vi "Error Handler.vi"() -> ()   [LabVIEW 2019]
uses:
  <vilib>/Utility/error.llb/Error Cluster From Error Code.vi
  <vilib>/ErrorRing/Error Ring.xnode
panel:
  in  "error in (no error)":errorcluster
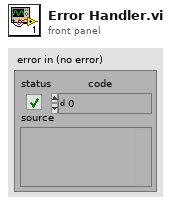
[diagram p1: front panel]
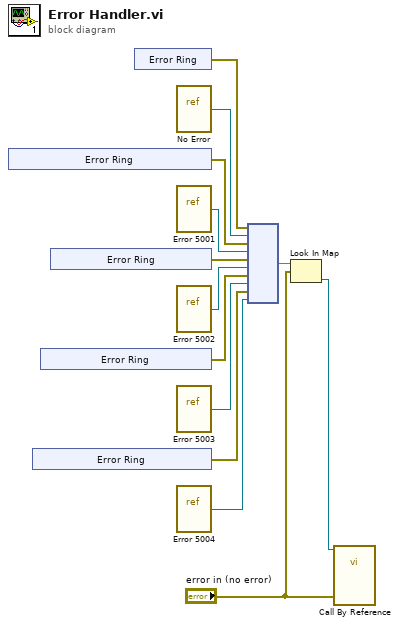
[diagram p0: block diagram]
diagram:
  n1 = xnode "Error Ring"() -> ("error out"=w12:errorcluster)
  n2 = xnode "Error Ring"() -> ("error out"=w6:errorcluster)
  n3 = xnode "Error Ring"() -> ("error out"=w8:errorcluster)
  n4 = xnode "Error Ring"() -> ("error out"=w11:errorcluster)
  n5 = xnode "Error Ring"() -> ("error out"=w13:errorcluster)
  n6 = vi-ref "No Error.vi"() -> (w3:refnum<vi>)
  n7 = vi-ref "Error 5001.vi"() -> (w10:refnum<vi>)
  n8 = vi-ref "Error 5002.vi"() -> (w9:refnum<vi>)
  n9 = vi-ref "Error 5003.vi"() -> (w7:refnum<vi>)
  n10 = vi-ref "Error 5004.vi"() -> (w5:refnum<vi>)
  n11 = node(w13, w3, w12, w10, w11, w9, w8, w7, w6, w5) -> (w4:map{errorcluster, refnum<vi>})
  n12 = Look In Map(map=w4, key="error in (no error)") -> (value=w2:refnum<vi>)  [unwired: 1 in, 1 out]
  n13 = call-by-ref "?"(reference=w2, "error in (no error)"="error in (no error)") -> ()  [unwired: 11 in, 3 out]
